vi "ILA_use.vi"() -> ()   [LabVIEW 2017]
panel:
  in  "String":string
  in  "ILA":bool
  in  "address":string="192.168.10.35"
  in  "error in (no error)":errorcluster
  out "error out":errorcluster
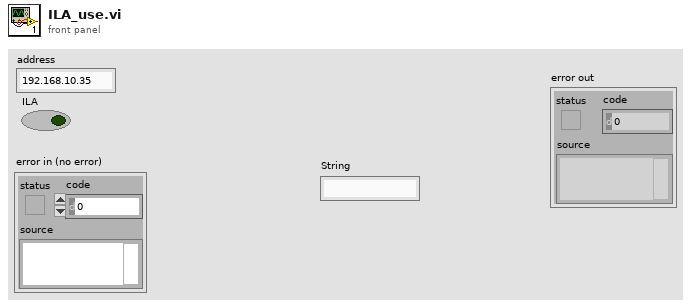
[diagram p1: front panel]
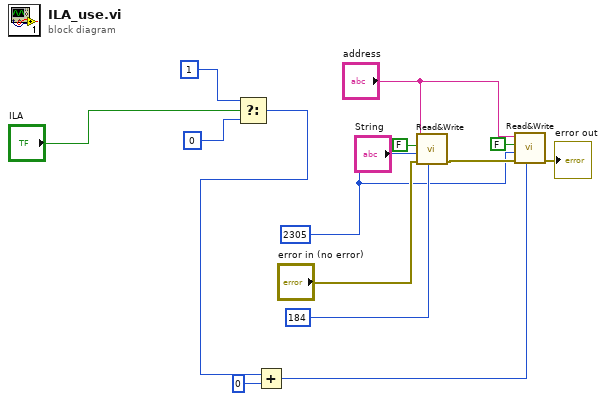
[diagram p0: block diagram]
diagram:
  w7 = u32 2305 ("Address")
  n1 = Select(t=u8 1 ("In 3"), s="ILA", f=u8 0 ("In 3")) -> (s? t:f=w3:u8)
  n2 = Add(x=w3, y=u8 0) -> (x+y=w4:u8)
  n3 = call "Read&Write.vi"("In"=u8 184, "error in (no error)"="error in (no error)", "Address"=w7, "Read (TRUE)"=FALSE, "address"="address") -> ("error out"=w14:errorcluster)  [unwired: 5 in, 1 out]
  n4 = call "Read&Write.vi"("In"=w4, "error in (no error)"=w14, "Address"=w7, "Read (TRUE)"=FALSE, "address"="address") -> ("error out"=→"error out":errorcluster)  [unwired: 5 in, 1 out]
